vi "DSF.Engine.Transceiver Thread.Main.vi"(8 "error in (no error)":errorcluster, 11 "Transceiver Thread in":refnum<class "DSF.Engine.Transceiver Thread.lvclass">) -> (0 "error out":errorcluster, 3 "Transceiver Thread out":refnum<class "DSF.Engine.Transceiver Thread.lvclass">)   [LabVIEW 2017, in "DSF.Engine.lvlib" / "DSF.Engine.Transceiver Thread.lvclass"]
uses:
  DSF.Engine.Transceiver Thread.lvclass
  DSF.Engine.Transceiver Thread.lvclass/DSF.Engine.Transceiver Thread.ctl
  Thread Parameters/Thread Parameters.lvclass/Thread Parameters.ctl
  <vilib>/Platform/TimedLoop/XDataNode/timing_clust.ctl
  <vilib>/Platform/TimedLoop/XDataNode/nitl_modes.ctl
  <vilib>/Platform/TimedLoop/XDataNode/wakeup.ctl
  Interface/DSF.Engine.Interface.lvclass/DSF.Engine.Interface.ctl
  Debug/DSF.Engine.Debug Flags.FIFO.lvclass/DSF.Engine.Debug Flags.FIFO.ctl
  Cache/DSF.Engine.Memory.Cache.lvclass/DSF.Engine.Memory.Cache.ctl
  Transfer/DSF.Engine.Transfer Group.lvclass/DSF.Engine.Transfer Group.ctl
  Timing/DSF.Engine.Timing.lvclass/DSF.Engine.Timing.ctl
  Debug/DSF.Engine.Debug Flags.lvclass/DSF.Engine.Debug Flags.ctl
  Thread Pool/DSF.Engine.Pool.lvclass/DSF.Engine.Pool.ctl
  Transfer/DSF.Engine.Transfer.lvclass/DSF.Engine.Transfer.ctl
  Pointer/DSF.Engine.Pointer.DBL.lvclass/DSF.Engine.Pointer.DBL.ctl
  <vilib>/National Instruments/Memory Manager/Classes/Pointer/Memory.Pointer.lvclass/Memory.Pointer.ctl
  Interface/DSF.Engine.Interface.Transceiver.Read.vi
  Interface/DSF.Engine.Interface.Transceiver.Read.Command.vi
  DSF.Engine.Transceiver Thread.Get Interface.vi
  DSF.Engine.Transceiver.Command.Cast.Transfer Group.To.vi
  DSF.Engine.Transceiver Thread.Transfer Group.Get by ID.vi
  Transfer/DSF.Engine.Transfer Group.Set Current Iteration.vi
  Transfer/DSF.Engine.Transfer Group.Return FIFO.Write.vi
  Thread Pool/DSF.Engine.Pool.ID.Return ID to Pool.vi
  DSF.Engine.Transceiver Thread.Get Thread ID Pool.vi
  Thread Parameters/Thread Parameters.Get ID.vi
  Transfer/DSF.Engine.Transfer Group.Get Transfers.vi
  DSF.Engine.Transceiver Thread.Transfer.Build.vi
  Interface/DSF.Engine.Interface.Read.Command.vi
  DSF.Engine.Transceiver Thread.Get Cache.vi
  Cache/DSF.Engine.Memory.Cache.Get Transfers Group.vi
  Transfer/DSF.Engine.Transfer Group.Get Timing.vi
  Timing/DSF.Engine.Timing.Iteration.Set.vi
  Transfer/DSF.Engine.Transfer Group.Set Timing.vi
  Transfer/DSF.Engine.Transfer Group.Get Return FIFO.vi
  Timing/DSF.Engine.Timing.Get Iteration.vi
  Transfer/DSF.Engine.Transfer Group.Get Debug Flags.vi
  Debug/DSF.Engine.Debug Flags.Get FIFO Flags.vi
  Debug/DSF.Engine.Debug Flags.FIFO.Get Infinite Timeouts.vi
  Thread Pool/DSF.Engine.Pool.Write FIFO.vi
  Buffer/DSF.Engine.Memory.Buffer.Insert Channels.Preserve Value.vi
  Transfer/DSF.Engine.Transfer.Get String Buffer.vi
  Transfer/DSF.Engine.Transfer.Get Intermediate Buffer.vi
  DSF.Engine.Transceiver Thread.Set Channels Buffer.vi
  DSF.Engine.Transceiver Thread.Get Channels Buffer.vi
  Transfer/DSF.Engine.Transfer.Get Channel Blocks.vi
  Pointer/DSF.Engine.Pointer.DBL.Read.vi
  Interface/DSF.Engine.Interface.Get Command FIFO.vi
  Interface/DSF.Engine.Interface.Get Debug Flags.vi
  Interface/DSF.Engine.Interface.RT FIFO.Read.16B.vi
  Cache/DSF.Engine.Memory.Cache.Get Transfers Groups.vi
  Timing/DSF.Engine.Timing.Set Iteration.vi
  Thread Pool/DSF.Engine.Pool.Get FIFO.vi
  Thread Pool/DSF.Engine.Pool.Get Debug Flags.vi
  <vilib>/National Instruments/Memory Manager/Classes/Pointer/Memory.Pointer.Read.vi
  <vilib>/National Instruments/Memory Manager/Classes/Pointer/Memory.Pointer.Read.1D.DBL.vi
  Pointer/DSF.Engine.Pointer.DBL.Get Channel Count.vi
  <vilib>/National Instruments/Memory Manager/Classes/Pointer/Memory.Pointer.Read.No Check.1D.DBL.vi
  <vilib>/National Instruments/Memory Manager/Classes/Pointer/Memory.Pointer.Parameter Check.Null Pointer.vi
  <vilib>/National Instruments/Memory Manager/Classes/Pointer/Memory.Pointer.Parameter Check.Subset.Power of 2.vi
  <vilib>/National Instruments/Memory Manager/Classes/Pointer/Memory.Pointer.Get Address.vi
  <vilib>/National Instruments/Memory Manager/Classes/Pointer/Memory.Pointer.Errors.vi
  <vilib>/National Instruments/Memory Manager/Classes/Pointer/Memory.Pointer.Errors.Null Pointer.vi
  <vilib>/National Instruments/Memory Manager/Classes/Pointer/Memory.Pointer.Errors.Out of Bounds.vi
  <vilib>/National Instruments/Memory Manager/Classes/Pointer/Memory.Pointer.Get Size.vi
  <vilib>/National Instruments/Memory Manager/Classes/Pointer/Memory.Pointer.Count to Size.Power of 2.vi
  <vilib>/National Instruments/Memory Manager/Classes/Pointer/Memory.Pointer.Errors.Create Error.vi
  <vilib>/NI/Static Error Handling/VIs/Static Error Handling.Source Buffer.Write.String.vi
  <vilib>/National Instruments/Memory Manager/Classes/Pointer/Memory.Pointer.Errors.Write Pointer Size.vi
  <vilib>/NI/Static Error Handling/VIs/Static Error Handling.Source Buffer.Write.Numeric.Scalar.Base10.vi
  <vilib>/NI/Static Error Handling/VIs/Static Error Handling.Source Buffer.Write.Numeric.Scalar.Base10 (U64).vi
  <vilib>/NI/Static Error Handling/VIs/Static Error Handling.Error Cluster Constant.vi
  <vilib>/NI/Static Error Handling/VIs/Static Error Handling.Error Cluster Constant (512B).vi
  <vilib>/NI/Static Error Handling/VIs/Static Error Handling.Parameters.Status.Set.vi
  <vilib>/NI/Static Error Handling/VIs/Static Error Handling.Parameters.Code.Set.vi
  <vilib>/NI/Static Error Handling/VIs/Static Error Handling.Parameters.VI Source.Set.vi
  <vilib>/National Instruments/Memory Manager/Constants/Memory.Constants.vi
  <vilib>/National Instruments/Memory Manager/Constants/Memory.Constants.Library Name.vi
  <vilib>/National Instruments/Memory Manager/Classes/Pointer/Memory.Pointer.Errors.Get Info.vi
  Interface/DSF.Engine.Interface.Transceiver.lvclass
  C:/Git/DSF/Source/Engine/Classes/Interface/DSF.Engine.Interface.lvclass
  Thread Pool/DSF.Engine.Pool.ID.lvclass
  C:/Git/DSF/Source/Engine/Classes/Thread Pool/DSF.Engine.Pool.lvclass
  Pointer/DSF.Engine.Pointer.DBL.lvclass
  C:/Program Files (x86)/National Instruments/LabVIEW 2017/vi.lib/National Instruments/Memory Manager/Classes/Pointer/Memory.Pointer.lvclass
  Buffer/DSF.Engine.Memory.Buffer.Write.vi
  Buffer/DSF.Engine.Memory.Buffer.Write.1D.Bool.vi
  Buffer/DSF.Engine.Memory.Buffer.Write.1D.SGL.vi
  Buffer/DSF.Engine.Memory.Buffer.Write.1D.DBL.vi
  Buffer/DSF.Engine.Memory.Buffer.Write.1D.I8.vi
  Buffer/DSF.Engine.Memory.Buffer.Write.1D.I16.vi
  Buffer/DSF.Engine.Memory.Buffer.Write.1D.I32.vi
  Buffer/DSF.Engine.Memory.Buffer.Write.1D.I64.vi
  Buffer/DSF.Engine.Memory.Buffer.Write.1D.U8.vi
  Buffer/DSF.Engine.Memory.Buffer.Write.1D.U16.vi
  Buffer/DSF.Engine.Memory.Buffer.Write.1D.U32.vi
  Buffer/DSF.Engine.Memory.Buffer.Write.1D.U64.vi
  <vilib>/platform/TimedLoop/XDataNode/XDataNode.xnode
  DSF.Engine.Transceiver.lvclass
  Thread Parameters/Thread Parameters.lvclass
  <vilib>/Platform/TimedLoop/XDataNode/XDNodeRunTimeDep.lvlib
panel:
  out "duration":u32
  out "iteration":i32
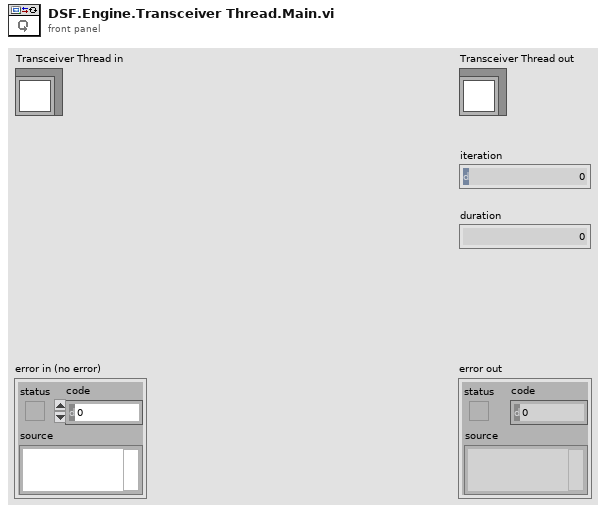
[diagram p1: front panel]
types:
  T1 = typedef "XDNodeRunTimeDep.lvlib/timing_clust.ctl" = cluster{"Expected End [f-1]":u64, "Actual End [f-1]":u64, "Finished Late? [f-1]":bool, "Expected End [i-1]":u64, "Actual End [i-1]":u64, "Finished Late? [i-1]":bool, "Expected Start [i]":u64, "Actual Start [i]":u64, "Expected Start [f]":u64, "Actual Start [f]":u64, "Source Name":string, "Structure Name":string, "Period":i64, "Deadline":i64, "Offset":i64, "Start":i64, "Priority":i32, "Timeout":i32, "Mode":T2, "Wakeup Reason":T3, "Error":errorcluster, "Source Type":string, "Secondary Source Type":string, "Global End Time":u64, "Global Start Time":u64, "Frame Duration":u64, "Iteration Duration":u64, "Assigned CPU":i32, "I/O Scan Engine Mode":u32}
  T2 = typedef "XDNodeRunTimeDep.lvlib/nitl_modes.ctl" = enum32{"No Change", "Process missed periods, maintain original phase", "Discard missed periods, maintain original phase", "Process missed periods, ignore original phase", "Discard missed periods, ignore original phase"}
  T3 = typedef "XDNodeRunTimeDep.lvlib/wakeup.ctl" = enum32{"Normal", "Aborted", "Asynchronous wakeup", "Timing source error", "Timed loop error", "Timeout"}
  T4 = typedef "DSF.Engine.lvlib/DSF.Engine.Interface.Transceiver.lvclass/DSF.Engine.Interface.Transceiver.Command Data.ctl" = cluster{"Command":T5, "Command Parameters":T6}
  T5 = typedef "DSF.Engine.lvlib/DSF.Engine.Interface.Transceiver.lvclass/DSF.Engine.Interface.Transceiver.Command.ctl" = enum8{"Rx", "Tx", "Shutdown"}
  T6 = typedef "DSF.Engine.lvlib/DSF.Engine.Interface.Transceiver.lvclass/DSF.Engine.Interface.Transceiver.Command Parameters.ctl" = cluster{"arg1":u64, "arg2":u64}
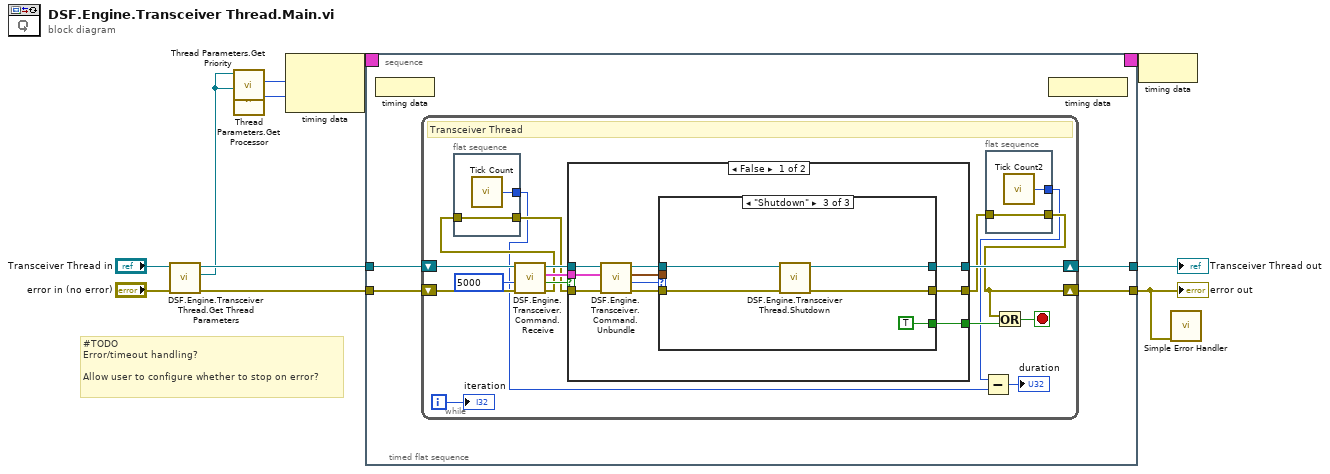
[diagram p0: block diagram]
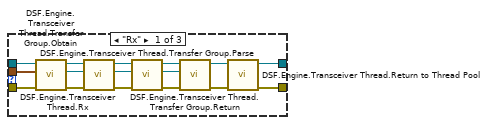
[diagram p2: hidden frame]
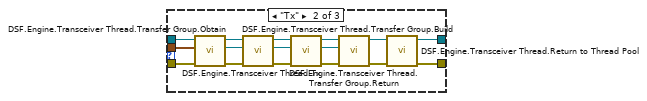
[diagram p3: hidden frame]
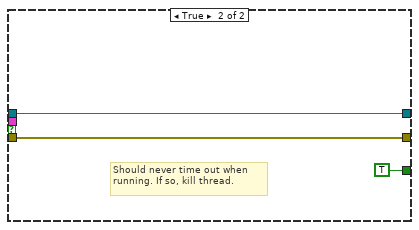
[diagram p4: hidden frame]
diagram:
  # "#TODO\nError/timeout handling?\n\nAllow user to configure whether to stop on error?"
  n1 = call "DSF.Engine.Transceiver Thread.Get Thread Parameters.vi"("Transceiver Thread in"="Transceiver Thread in") -> ("Thread Parameters"=w3:refnum<class "Thread Parameters.lvclass">, "Transceiver Thread out"=w4:refnum<class "DSF.Engine.Transceiver Thread.lvclass">)  [unwired: 9 in]
  n2 = call "Thread Parameters.Get Priority.vi"("Thread Parameters in"=w3) -> ("Priority"=w6:i32)  [unwired: 9 in, 1 out]
  n3 = call "Thread Parameters.Get Processor.vi"("Thread Parameters in"=w3) -> ("Processor"=w5:i32)  [unwired: 9 in, 1 out]
  n4 = node-c288(w6, w5) -> (w10:T1)
  n5 = timed-sequence {
    timing: w10 -> [_]
    timing-out: [_] -> w9
    tunnel: w4 -> [w14]
    tunnel: [w13] -> w8
    tunnel: "error in (no error)" -> [w12]
    tunnel: [w11] -> w1
    n6 = timed-flat-sequence {
      tunnel: w14 -> [w18]
      tunnel: [w17] -> w13
      tunnel: w12 -> [w16]
      tunnel: [w15] -> w11
      n7 = node-c288() -> ()  [unwired: 1 in]
      n8 = while {
        shift-right: [w22] -> w15
        shift-left: w16 -> [w33]
        shift-right: [w29] -> w17
        shift-left: w18 -> [w30]
        i -> [w26]
        stop <- w27 stop-if-true
        # "Transceiver Thread"
        n9 = flat-sequence {
          tunnel: [w39] -> w24
          tunnel: w25 -> [w39]
          tunnel: [w38] -> w20
          frame #0 {
            n10 = call "Tick Count"() -> ("Tick Count(uSec)"=w38:u32)
          }
        }
        n11 = call "DSF.Engine.Transceiver.Command.Receive.vi"("error in (no error)"=w33, "timeout in ms (0)"=5000 ("timeout in ms"), "Transceiver Thread in"=w30) -> ("error out"=w25:errorcluster, "timed out?"=w31:bool, "command"=w32:T4, "Transceiver Thread out"=w34:refnum<class "DSF.Engine.Transceiver Thread.lvclass">)  [unwired: 5 in]
        n12 = case shown="False" w31 {
          tunnel: w34 -> [w46 w88]
          tunnel: [w49 w88] -> w29
          tunnel: w24 -> [w45 w87]
          tunnel: w32 -> [w44 _]
          tunnel: [w48 w87] -> w23
          tunnel: [w47 TRUE] -> w28
          frame False {
            n13 = call "DSF.Engine.Transceiver.Command.Unbundle.vi"("error in (no error)"=w45, "command"=w44, "Transceiver Thread in"=w46) -> ("error out"=w42:errorcluster, "command"=w43:T5, "command parameters"=w40:T6, "Transceiver Thread out"=w41:refnum<class "DSF.Engine.Transceiver Thread.lvclass">)  [unwired: 5 in]
            n14 = case shown="\"Shutdown\"" w43 {
              tunnel: w41 -> [w55 w71 w85]
              tunnel: [w57 w74 w83] -> w49
              tunnel: w42 -> [w50 w70 w84]
              tunnel: w40 -> [w54 w67 _]
              tunnel: [w56 w73 w82] -> w48
              tunnel: [_ _ TRUE] -> w47
              frame "Rx" {
                n15 = call "DSF.Engine.Transceiver Thread.Transfer Group.Obtain.vi"("error in (no error)"=w50, "command parameters"=w54, "Transceiver Thread in"=w55) -> ("error out"=w52:errorcluster, "Transfer Group"=w51:refnum<class "DSF.Engine.Transfer Group.lvclass">, "Transceiver Thread out"=w53:refnum<class "DSF.Engine.Transceiver Thread.lvclass">)  [unwired: 6 in]
                n16 = call "DSF.Engine.Transceiver Thread.Rx.vi"("error in (no error)"=w52, "Transfer Group in"=w51, "Transceiver Thread in"=w53) -> ("error out"=w64:errorcluster, "Transfer Group out"=w63:refnum<class "DSF.Engine.Transfer Group.lvclass">, "Transceiver Thread out"=w65:refnum<class "DSF.Engine.Transceiver Thread.lvclass">)  [unwired: 6 in]
                n17 = call "DSF.Engine.Transceiver Thread.Transfer Group.Parse.vi"("error in (no error)"=w64, "Transfer Group in"=w63, "Transceiver Thread in"=w65) -> ("error out"=w61:errorcluster, "Transfer Group out"=w60:refnum<class "DSF.Engine.Transfer Group.lvclass">, "Transceiver Thread out"=w62:refnum<class "DSF.Engine.Transceiver Thread.lvclass">)  [unwired: 6 in]
                n18 = call "DSF.Engine.Transceiver Thread.Transfer Group.Return.vi"("error in (no error)"=w61, "Transfer Group"=w60, "Transceiver Thread in"=w62) -> ("error out"=w58:errorcluster, "Transceiver Thread out"=w59:refnum<class "DSF.Engine.Transceiver Thread.lvclass">)  [unwired: 7 in]
                n19 = call "DSF.Engine.Transceiver Thread.Return to Thread Pool.vi"("error in (no error)"=w58, "Transceiver Thread in"=w59) -> ("error out"=w56:errorcluster, "Transceiver Thread out"=w57:refnum<class "DSF.Engine.Transceiver Thread.lvclass">)  [unwired: 8 in]
              }
              frame "Tx" {
                n20 = call "DSF.Engine.Transceiver Thread.Transfer Group.Obtain.vi"("error in (no error)"=w70, "command parameters"=w67, "Transceiver Thread in"=w71) -> ("error out"=w68:errorcluster, "Transfer Group"=w66:refnum<class "DSF.Engine.Transfer Group.lvclass">, "Transceiver Thread out"=w69:refnum<class "DSF.Engine.Transceiver Thread.lvclass">)  [unwired: 6 in]
                n21 = call "DSF.Engine.Transceiver Thread.Transfer Group.Build.vi"("error in (no error)"=w68, "Transfer Group in"=w66, "Transceiver Thread in"=w69) -> ("error out"=w80:errorcluster, "Transfer Group out"=w72:refnum<class "DSF.Engine.Transfer Group.lvclass">, "Transceiver Thread out"=w81:refnum<class "DSF.Engine.Transceiver Thread.lvclass">)  [unwired: 6 in]
                n22 = call "DSF.Engine.Transceiver Thread.Tx.vi"("error in (no error)"=w80, "Transfer Group in"=w72, "Transceiver Thread in"=w81) -> ("error out"=w78:errorcluster, "Transfer Group out"=w77:refnum<class "DSF.Engine.Transfer Group.lvclass">, "Transceiver Thread out"=w79:refnum<class "DSF.Engine.Transceiver Thread.lvclass">)  [unwired: 6 in]
                n23 = call "DSF.Engine.Transceiver Thread.Transfer Group.Return.vi"("error in (no error)"=w78, "Transfer Group"=w77, "Transceiver Thread in"=w79) -> ("error out"=w75:errorcluster, "Transceiver Thread out"=w76:refnum<class "DSF.Engine.Transceiver Thread.lvclass">)  [unwired: 7 in]
                n24 = call "DSF.Engine.Transceiver Thread.Return to Thread Pool.vi"("error in (no error)"=w75, "Transceiver Thread in"=w76) -> ("error out"=w73:errorcluster, "Transceiver Thread out"=w74:refnum<class "DSF.Engine.Transceiver Thread.lvclass">)  [unwired: 8 in]
              }
              frame "Shutdown" {
                n25 = call "DSF.Engine.Transceiver Thread.Shutdown.vi"("error in (no error)"=w84, "Transceiver Thread in"=w85) -> ("error out"=w82:errorcluster, "Transceiver Thread out"=w83:refnum<class "DSF.Engine.Transceiver Thread.lvclass">)  [unwired: 8 in]
              }
            }
          }
          frame True {
            # "Should never time out when running. If so, kill thread."
          }
        }
        n26 = Subtract(x=w21, y=w20) -> (x-y=→"duration":u32)
        n27 = flat-sequence {
          tunnel: [w37] -> w22
          tunnel: w23 -> [w37]
          tunnel: [w36] -> w21
          frame #0 {
            n28 = call "Tick Count2"() -> ("Tick Count(uSec)"=w36:u32)
          }
        }
        n29 = Or(x=w22, y=w28) -> (x .or. y?=w27:bool)
        "iteration" <- w26
      }
      n30 = node-c288() -> ()  [unwired: 1 out]
    }
  }
  "error out" <- w1
  "Transceiver Thread out" <- w8
  n31 = node-c288(w9) -> ()
  n32 = call <vilib>:"Simple Error Handler.vi"("error in (no error)"=w1) -> ()  [unwired: 4 in, 5 out]
